vi "Odczyt azymutu z odometrii.vi"(6 "Reset":T1, 7 "Azymut robota\n pocz/nowy":dbl caption="Azymut robota pocz/nowy" min=0.0 max=360.0, 9 "Położenie bazy":T3, 10 "Parametry odwzorowania Ziemi (WGS84)":cluster{"a":dbl, "b":dbl}={"a"=6378137.0, "b"=6356752.3142} {"b" format="%#.6g"; "a" format="%#.6g"}, 11 "Ustawienia początkowe":T2) -> (1 "Azymut [stopnie]":dbl, 2 "Odczyt GPS":T4, 3 "Odległość robota od bazy [m]":cluster{"X [m]":dbl, "Y [m]":dbl})   [LabVIEW 2015, in "Biblioteka moduł map v3.lvlib" / "Pomocnicze.lvlib"]
uses:
  Pomocnicze/Pomocnicze.lvlib
  Zmienne/Lokalizacja GPS/azymut.vi
  Zmienne/szablon odometry_filtered_local.vi
  Matematyczne/Matematyczne.lvlib
  Zmienne/Zmienne.lvlib
  TASK ERL/task erl.lvlib
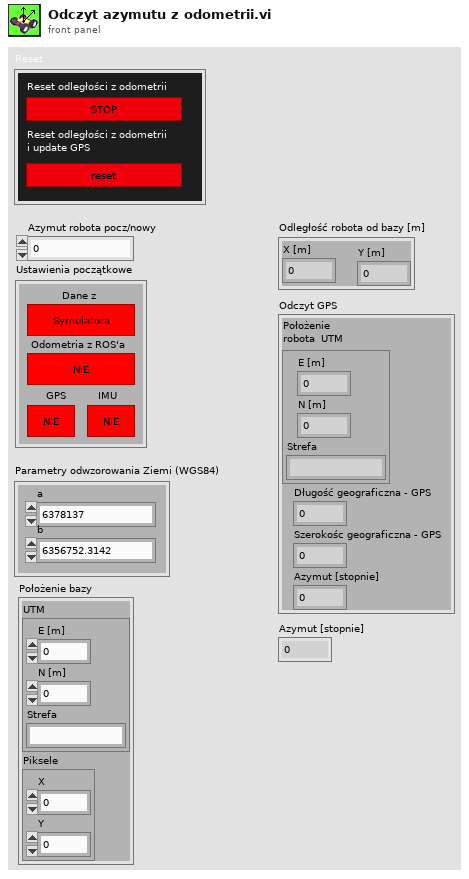
[diagram p1: front panel]
types:
  T1 = cluster{"reset odom":bool, "reset odom + gps":bool}
  T2 = cluster{"Dane z":bool, "Odometria z ROS'a":bool, "GPS":bool, "IMU":bool}
  T3 = cluster{"UTM":cluster{"E [m]":dbl, "N [m]":dbl, "Strefa":string}, "Piksele":cluster{"X":i32, "Y":i32}}
  T4 = cluster{"Położenie \nrobota  UTM":cluster{"E [m]":ext, "N [m]":ext, "Strefa":string}, "Długość geograficzna - GPS":dbl, "Szerokośc geograficzna - GPS":dbl, "Azymut [stopnie]":dbl}
  T5 = typedef "Biblioteka moduł map v3.lvlib/Zmienne.lvlib/szablon odometry_filtered_local.ctl" = cluster{"topic":string, "msg":cluster{"header":cluster{"seq":u32, "stamp":cluster{"secs":u32, "nsecs":i32}, "frame_id":string}, "child_frame_id":string, "pose":cluster{"pose":cluster{"position":cluster{"y":dbl, "z":dbl, "x":dbl}, "orientation":cluster{"y":dbl, "z":dbl, "x":dbl, "w":dbl}}, "covariance":dbl[]}, "twist":cluster{"twist":cluster{"linear":cluster{"y":dbl, "z":dbl, "x":dbl}, "angular":cluster{"y":dbl, "z":dbl, "x":dbl}}, "covariance":dbl[]}}, "op":string}
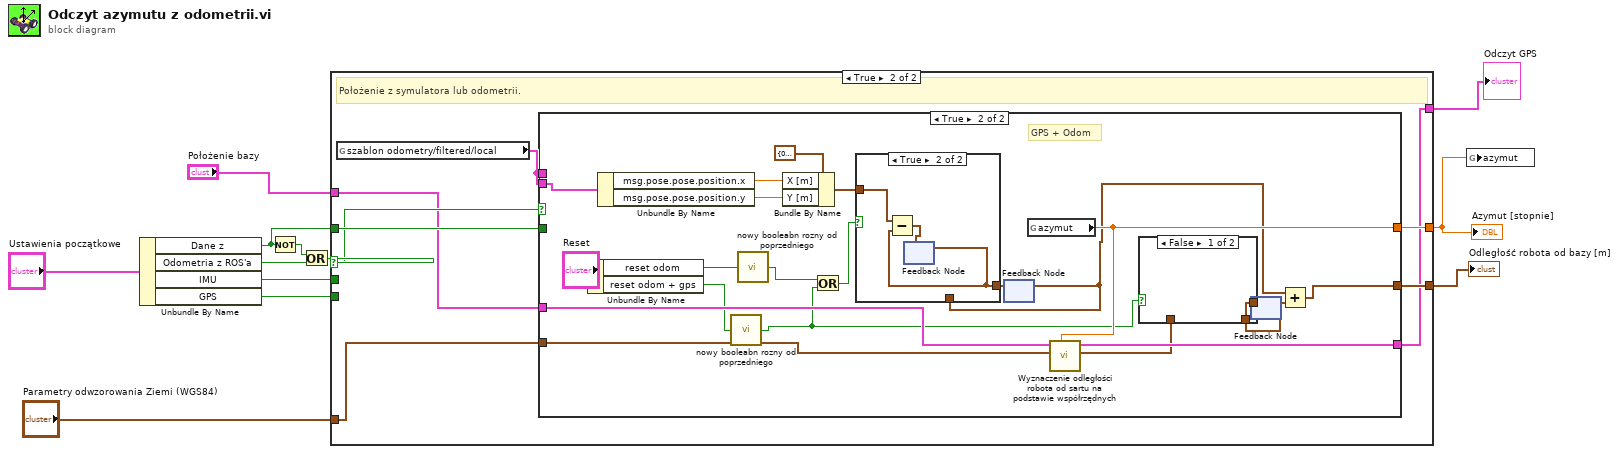
[diagram p0: block diagram]
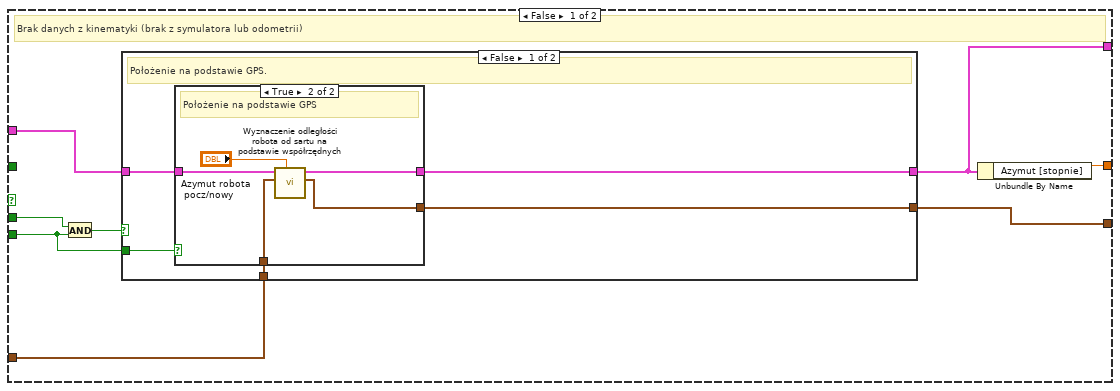
[diagram p2: hidden frame]
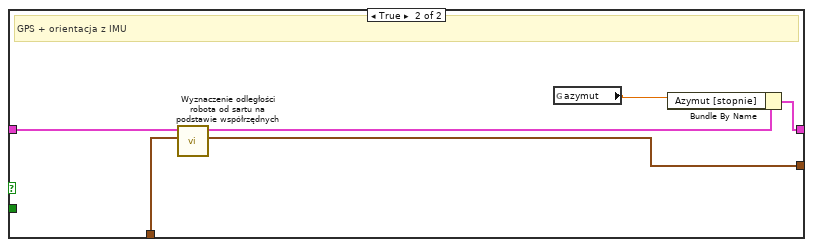
[diagram p4: hidden frame]
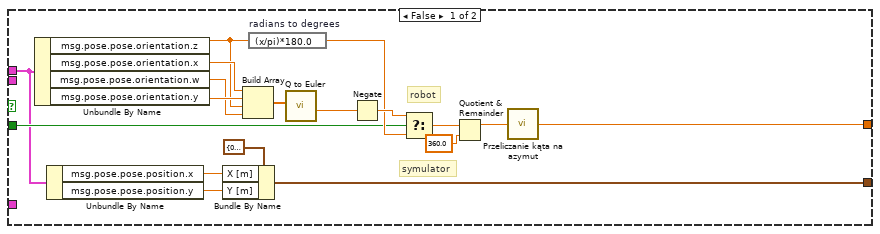
[diagram p5: hidden frame]
diagram:
  n1 = Unbundle By Name("Ustawienia początkowe") -> ("Dane z"=w8:bool, "Odometria z ROS'a"=w12:bool, "IMU"=w7:bool, "GPS"=w5:bool)
  n2 = Not(x=w8) -> (.not. x?=w9:bool)
  n3 = Or(x=w9, y=w12) -> (x .or. y?=w11:bool)
  n4 = case shown="True" w11 {
    selector: w11 -> [_ w41]
    tunnel: [w19 w44] -> w10
    tunnel: [w20 w42] -> w3
    tunnel: w8 -> [_ w43]
    tunnel: w7 -> [w18 _]
    tunnel: w5 -> [w16 _]
    tunnel: "Parametry odwzorowania Ziemi (WGS84)" -> [w15 w39]
    tunnel: [w14 w37] -> w2
    tunnel: "Położenie bazy" -> [w13 w38]
    frame False {
      # "Brak danych z kinematyki (brak z symulatora lub odometrii)"
      n5 = And(x=w18, y=w16) -> (x .and. y?=w17:bool)
      n6 = case shown="False" w17 {
        tunnel: w13 -> [w25 w36]
        tunnel: [w24 w33] -> w19
        tunnel: [w23 w34] -> w14
        tunnel: w15 -> [w22 w35]
        tunnel: w16 -> [w21 _]
        frame False {
          # "Położenie na podstawie GPS."
          n7 = case shown="True" w21 {
            tunnel: w25 -> [_ w30]
            tunnel: [_ w29] -> w24
            tunnel: [_ w27] -> w23
            tunnel: w22 -> [_ w26]
            frame False {
              # "brak możliwości ustalenia pozycji."
            }
            frame True {
              # "Położenie na podstawie GPS"
              n8 = call "Wyznaczenie odległości robota od sartu na podstawie współrzędnych.vi"("Azymut robota\n pocz/nowy"="Azymut robota\n pocz/nowy", "Parametry odwzorowania Ziemi (WGS84)"=w26, "Pocz. poł."=w30) -> ("Rzeczywista odległość robota od startu [m]"=w29:cluster{"X [m]":dbl, "Y [m]":dbl}, "Aktualne położenie"=w27:T4)  [unwired: 7 in]
            }
          }
        }
        frame True {
          # "GPS + orientacja z IMU"
          n9 = call "Wyznaczenie odległości robota od sartu na podstawie współrzędnych.vi"("Parametry odwzorowania Ziemi (WGS84)"=w35, "Pocz. poł."=w36) -> ("Rzeczywista odległość robota od startu [m]"=w33:cluster{"X [m]":dbl, "Y [m]":dbl}, "Aktualne położenie"=w32:T4)  [unwired: 8 in]
          n10 = global read "azymut.vi" "azymut"() -> (w31:dbl)
          n11 = Bundle By Name(cluster=w32, "Azymut [stopnie]"=w31) -> (w34:T4)
        }
      }
      n12 = Unbundle By Name(w14) -> ("Azymut [stopnie]"=w20:dbl)
    }
    frame True {
      # "Położenie z symulatora lub odometrii."
      n13 = global read "szablon odometry_filtered_local.vi" "szablon odometry/filtered/local"() -> (w40:T5)
      n14 = case shown="True" w41 {
        tunnel: [w59 w64] -> w44
        tunnel: w43 -> [w47 _]
        tunnel: [w46 w73] -> w42
        tunnel: w40 -> [w45 _]
        tunnel: w40 -> [_ w83]
        tunnel: w39 -> [_ w75]
        tunnel: w38 -> [_ w74]
        tunnel: [_ w72] -> w37
        frame False {
          # "symulator"
          # "robot"
          n15 = Unbundle By Name(w45) -> ("msg.pose.pose.orientation.z"=w49:dbl, "msg.pose.pose.orientation.x"=w57:dbl, "msg.pose.pose.orientation.w"=w55:dbl, "msg.pose.pose.orientation.y"=w56:dbl)
          n16 = Unbundle By Name(w45) -> ("msg.pose.pose.position.x"=w61:dbl, "msg.pose.pose.position.y"=w62:dbl)
          n17 = Bundle By Name(cluster=cluster{"X [m]":dbl, "Y [m]":dbl} {"X [m]"=0.0, "Y [m]"=0.0} ("Odległość robota od startu [m]"), "X [m]"=w61, "Y [m]"=w62) -> (w59:cluster{"X [m]":dbl, "Y [m]":dbl})
          n18 = Build Array(w57, w56, w49, w55) -> (w54:dbl[])
          n19 = expression code="(x/pi)*180.0" "radians to degrees"(w49) -> (w48:dbl)
          n20 = call "Q to Euler.vi"("array"=w54) -> ("Yaw"=w52:dbl)  [unwired: 3 in, 3 out]
          n21 = Negate(x=w52) -> (-x=w51:dbl)
          n22 = Select(t=w51, s=w47, f=w48) -> (s? t:f=w50:dbl)
          n23 = Quotient & Remainder(x=w50, y=360.0) -> (x-y*floor(x/y)=w53:dbl)  [unwired: 1 out]
          n24 = call "Przeliczanie kąta na azymut.vi"("Kąt [stoponie]"=w53) -> ("Azymut [stopnie]"=w46:dbl)  [unwired: 4 in]
        }
        frame True {
          # "GPS + Odom"
          n25 = Unbundle By Name("Reset") -> ("reset odom"=w77:bool, "reset odom + gps"=w69:bool)
          n26 = Unbundle By Name(w83) -> ("msg.pose.pose.position.x"=w81:dbl, "msg.pose.pose.position.y"=w80:dbl)
          n27 = call "nowy booleabn rozny od poprzedniego.vi"("Boolean"=w69) -> ("x != y?"=w63:bool)  [unwired: 4 in]
          n28 = call "nowy booleabn rozny od poprzedniego.vi"("Boolean"=w77) -> ("x != y?"=w70:bool)  [unwired: 4 in]
          n29 = Bundle By Name(cluster=cluster{"X [m]":dbl, "Y [m]":dbl} {"X [m]"=0.0, "Y [m]"=0.0} ("Odległość robota od startu [m]"), "X [m]"=w81, "Y [m]"=w80) -> (w78:cluster{"X [m]":dbl, "Y [m]":dbl})
          n30 = Or(x=w70, y=w63) -> (x .or. y?=w68:bool)
          n31 = feedback #1() -> (w67:cluster{"X [m]":dbl, "Y [m]":dbl})  [unwired: 1 in]
          n32 = case shown="True" w68 {
            tunnel: w78 -> [_ w89]
            tunnel: [w86 w87] -> w76
            tunnel: w67 -> [w86 _]
            frame False {
            }
            frame True {
              n33 = feedback #2() -> (w87:cluster{"X [m]":dbl, "Y [m]":dbl})  [unwired: 1 in]
              n34 = Subtract(x=w89, y=w87) -> (x-y=w88:cluster{"X [m]":dbl, "Y [m]":dbl})
              n35 = feedback-in #2(w88) -> ()
            }
          }
          n36 = feedback-in #1(w76) -> ()
          n37 = global read "azymut.vi" "azymut"() -> (w73:dbl)
          n38 = call "Wyznaczenie odległości robota od sartu na podstawie współrzędnych.vi"("Azymut robota\n pocz/nowy"=w73, "Parametry odwzorowania Ziemi (WGS84)"=w75, "Pocz. poł."=w74) -> ("Rzeczywista odległość robota od startu [m]"=w71:cluster{"X [m]":dbl, "Y [m]":dbl}, "Aktualne położenie"=w72:T4)  [unwired: 7 in]
          n39 = feedback #3() -> (w65:cluster{"X [m]":dbl, "Y [m]":dbl})  [unwired: 1 in]
          n40 = case shown="False" w63 {
            tunnel: w71 -> [_ w85]
            tunnel: [w84 w85] -> w66
            tunnel: w65 -> [w84 _]
            frame False {
            }
            frame True {
            }
          }
          n41 = feedback-in #3(w66) -> ()
          n42 = Add(x=w67, y=w65) -> (x+y=w64:cluster{"X [m]":dbl, "Y [m]":dbl})
        }
      }
    }
  }
  "Azymut [stopnie]" <- w3
  "Odległość robota od bazy [m]" <- w10
  "Odczyt GPS" <- w2
  n43 = global write "azymut.vi" "azymut"(w3) -> ()
